vi "TraverseStateMain.vi"(8 "error in (no error)":errorcluster, 10 "SelList[]":refnum<vi>[](array[refnum]), 11 "Vi Ref":refnum<vi>) -> (0 "error out":errorcluster)   [LabVIEW 2012]
uses:
  <vilib>/Utility/traverseref.llb/TRef TravTarget.ctl
  <vilib>/Utility/traverseref.llb/VI Scripting - Traverse.lvlib
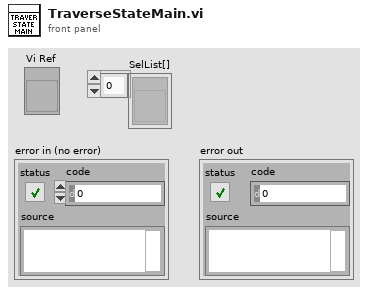
[diagram p1: front panel]
types:
  T1 = typedef "TRef TravTarget.ctl" = enum16{"FP", "BD", "Other"}
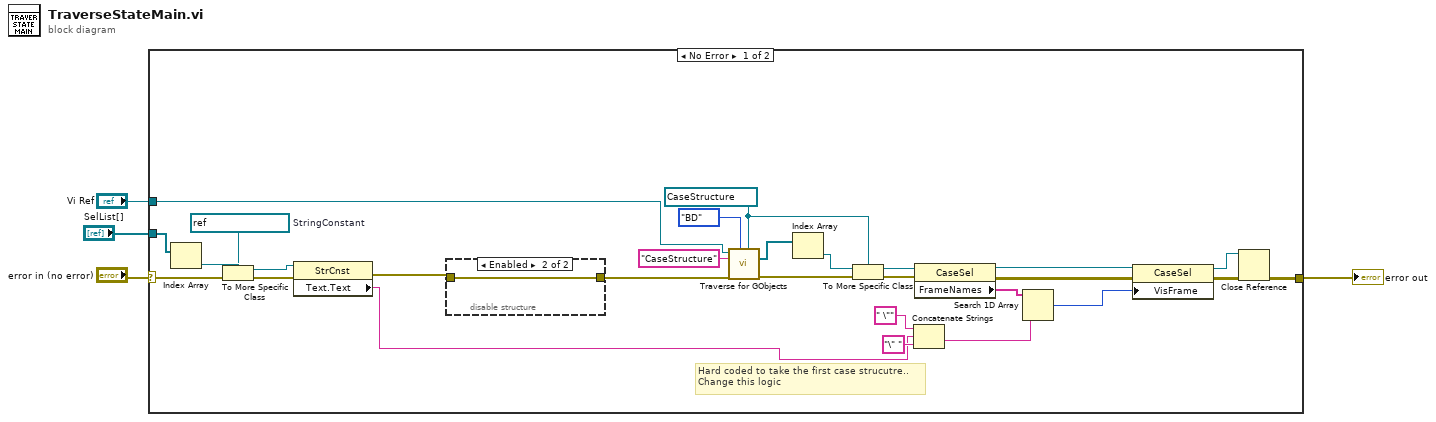
[diagram p0: block diagram]
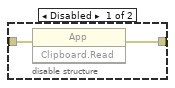
[diagram p2: hidden frame]
diagram:
  n1 = case shown="No Error" "error in (no error)" {
    selector: "error in (no error)" -> [w6 w36]
    tunnel: [w20 w36] -> w3
    tunnel: "Vi Ref" -> [w31 _]
    tunnel: "SelList[]" -> [w12 _]
    frame No Error {
      w10 = refnum<vi> refnum  # StringConstant
      w24 = refnum<vi> refnum ("Other Refnum")
      # "Hard coded to take the first case strucutre..\nChange this logic"
      n2 = Index Array(array=w12) -> (element=w11:refnum<vi>)  [unwired: 1 in]
      n3 = To More Specific Class(target class=w10, reference=w11, error in=w6) -> (specific class reference=w9:refnum<vi>, error out=w7:errorcluster)
      n4 = property class="StrCnst"(reference=w9, error in=w7) -> (error out=w5:errorcluster, "Text.Text"=w8:string)  [unwired: 1 out]
      n5 = disable-structure shown="Enabled" {
        disable-tunnel: [w34 w35] -> w15
        disable-tunnel: w5 -> [w33 w35]
        frame Disabled {
          n6 = invoke class="App" method="Clipboard.Read"(error in=w33) -> (error out=w34:errorcluster)  [unwired: 2 in, 2 out]
        }
        frame Enabled {
        }
      }
      n7 = call <vilib>:"Traverse for GObjects.vi"("Other Refnum"=w24, "Traverse Target"=TRef_TravTarget."BD", "error in (no error)"=w15, "Class Name"="CaseStructure", "VI Refnum"=w31) -> ("error out"=w32:errorcluster, "References"=w28:refnum<vi>[])  [unwired: 3 in, 2 out]
      n8 = Index Array(array=w28) -> (element=w26:refnum<vi>)  [unwired: 1 in]
      n9 = To More Specific Class(target class=w24, reference=w26, error in=w32) -> (specific class reference=w25:refnum<vi>, error out=w27:errorcluster)
      n10 = Concatenate Strings(" \"" ("string"), w8, "\" " ("string")) -> (w17:string)
      n11 = property class="CaseSel"(reference=w25, error in=w27) -> (reference out=w13:refnum<vi>, error out=w23:errorcluster, "FrameNames"=w18:string[])
      n12 = Search 1D Array(1D array=w18, element=w17) -> (index of element=w22:i32)  [unwired: 1 in]
      n13 = property class="CaseSel"(reference=w13, error in=w23, "VisFrame"=w22) -> (reference out=w19:refnum<vi>, error out=w21:errorcluster)
      n14 = Close Reference(reference=w19, error in (no error)=w21) -> (error out=w20:errorcluster)
    }
    frame Error {
    }
  }
  "error out" <- w3
